vi "img.rescaleProfile.vi"(6 "range":T1, 9 "MarkerVals in (greyscale)":cluster{dbl, u32}[](array[cluster])=[{0.0, 0}, {1.0, 16777215}] {"?" format="%06x"}) -> (1 "MarkerVals out":cluster{dbl, u32}[](array[cluster]) {"?" format="%06.0f"}, 4 "extrema":cluster{"high":u32, "low":u32})   [LabVIEW 2020]
uses:
  _controls/cluster.range.sgl.ctl
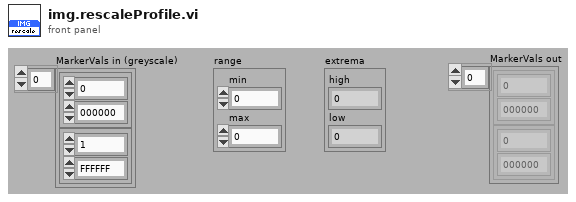
[diagram p1: front panel]
types:
  T1 = typedef "cluster.range.sgl.ctl" = cluster{"min":sgl, "max":sgl}
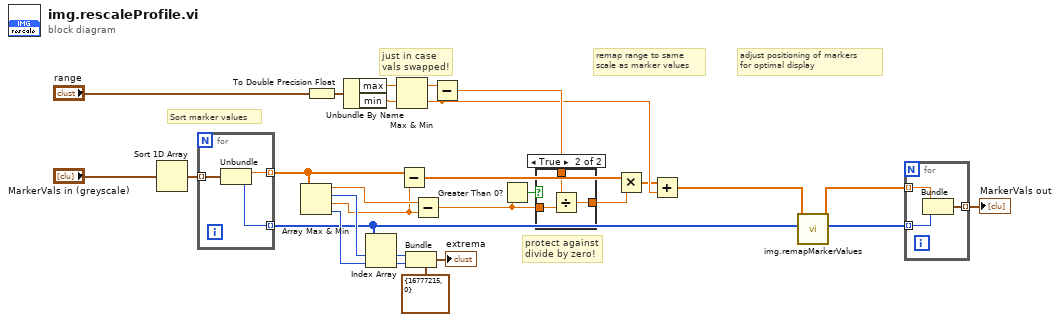
[diagram p0: block diagram]
diagram:
  # "Sort marker values"
  # "adjust positioning of markers \nfor optimal display"
  # "remap range to same\nscale as marker values"
  # "protect against \ndivide by zero!"
  # "just in case \nvals swapped!"
  n1 = Sort 1D Array(array="MarkerVals in (greyscale)") -> (sorted array=w4:cluster{dbl, u32}[])
  n2 = for {
    tunnel: w4 -> [w31] mode=indexing
    tunnel: [w30] -> w3 mode=indexing
    tunnel: [w29] -> w2 mode=indexing
    n3 = Unbundle(w31) -> (w30:dbl, w29:u32)
  }
  n4 = Array Max & Min(array=w3) -> (max value=w9:dbl, max index (indices)=w11:i32, min value=w8:dbl, min index (indices)=w10:i32)
  n5 = To Double Precision Float(number="range") -> (double precision float=w12:cluster{"min":dbl, "max":dbl})
  n6 = Unbundle By Name(w12) -> ("max"=w27:dbl, "min"=w26:dbl)
  n7 = Index Array(array=w2, index #1=w11, index #2=w10) -> (element #1=w20:u32, element #2=w19:u32)
  n8 = Max & Min(x=w27, y=w26) -> (max(x,y)=w25:dbl, min(x,y)=w22:dbl)
  n9 = Subtract(x=w3, y=w8) -> (x-y=w23:dbl[])
  n10 = Bundle(cluster=cluster{"high":u32, "low":u32} {"high"=16777215, "low"=0} ("extrema"), "high"=w20, "low"=w19) -> (→"extrema":cluster{"high":u32, "low":u32})
  n11 = Subtract(x=w9, y=w8) -> (x-y=w16:dbl)
  n12 = Subtract(x=w25, y=w22) -> (x-y=w24:dbl)
  n13 = Greater Than 0?(x=w16) -> (x > 0?=w13:bool)
  n14 = case shown="True" w13 {
    tunnel: w24 -> [_ w34]
    tunnel: w16 -> [_ w33]
    tunnel: [_ w32] -> w15
    frame False {
    }
    frame True {
      n15 = Divide(x=w34, y=w33) -> (x/y=w32:dbl)
    }
  }
  n16 = Multiply(x=w23, y=w15) -> (x*y=w14:dbl[])
  n17 = Add(x=w14, y=w22) -> (x+y=w7:dbl[])
  n18 = call "img.remapMarkerValues.vi"("colours in"=w2, "marker values in"=w7) -> ("colours out"=w5:u32[], "marker values out"=w6:dbl[])  [unwired: 1 in, 7 out]
  n19 = for {
    tunnel: w5 -> [w36] mode=indexing
    tunnel: w6 -> [w37] mode=indexing
    tunnel: [w35] -> w21 mode=indexing
    n20 = Bundle(w37, w36) -> (w35:cluster{dbl, u32})  [unwired: 1 out]
  }
  "MarkerVals out" <- w21
